vi "test Get-Set-Get AIM Hardware Parameters.vi"(8 "error in":errorcluster, 11 "TestCase in":refnum<class "Scripting.lvclass">) -> (0 "error out":errorcluster, 3 "TestCase out":refnum<class "Scripting.lvclass">)   [LabVIEW 2020, in "Scripting.lvclass"]
uses:
  Scripting.lvclass
  <vilib>/addons/_JKI Toolkits/VI Tester/TestCase.llb/TestCase.lvclass
  Scripting/AIM MIL-STD-1553 Scripting.lvlib
  Shared/Initialization Method.ctl
  Shared/AIM Hardware Parameters.ctl
  Shared/Coupling Mode.ctl
  Shared/Bus Selection.ctl
  Shared/Timing Mode.ctl
  C:/Program Files (x86)/National Instruments/LabVIEW 2020/vi.lib/addons/_JKI Toolkits/VI Tester/TestCase.llb/TestCase.lvclass
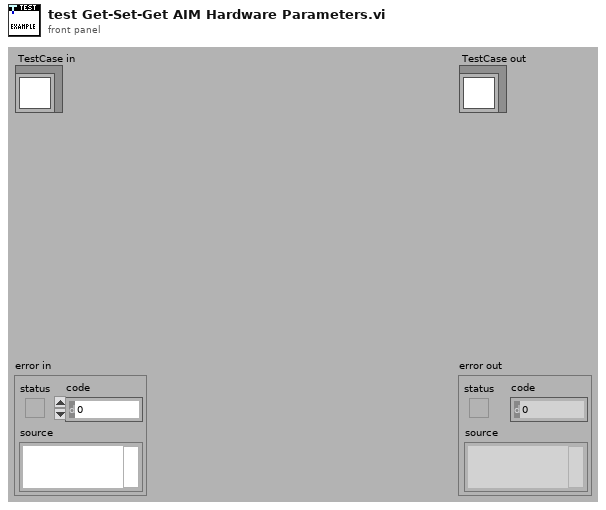
[diagram p1: front panel]
types:
  T1 = typedef "AIM Hardware Parameters.ctl" = cluster{"initialization method":T2, "card number":i32, "pxi slot number":i32, "biu number":i32, "bus selection":T3, "coupling mode":T4, "timing mode":T5}
  T2 = typedef "Initialization Method.ctl" = enum16{"PXI Slot Number", "Card Number"}
  T3 = typedef "Bus Selection.ctl" = enum16{"Both", "Primary", "Secondary"}
  T4 = typedef "Coupling Mode.ctl" = enum16{"Isolated Onboard Termination", "Transformer Coupled", "Direct Coupled", "External with Onboard Termination", "Onboard Digital Wrap-around"}
  T5 = typedef "Timing Mode.ctl" = enum16{"Disabled (Relative Timestamps)", "IRIG (Internal System Time)", "IRIG (External Timing Source)"}
  T6 = typedef "Custom Device API.lvlib/Custom Device Item Ref.ctl" = u64
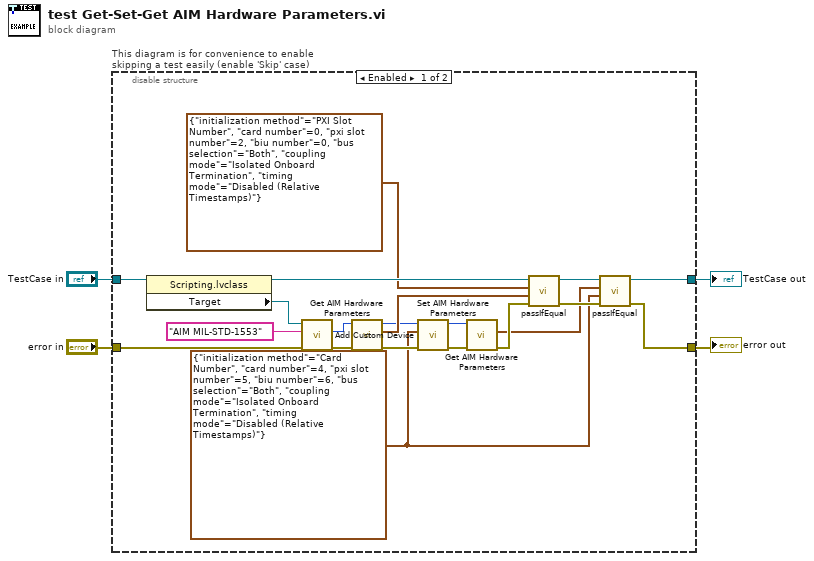
[diagram p0: block diagram]
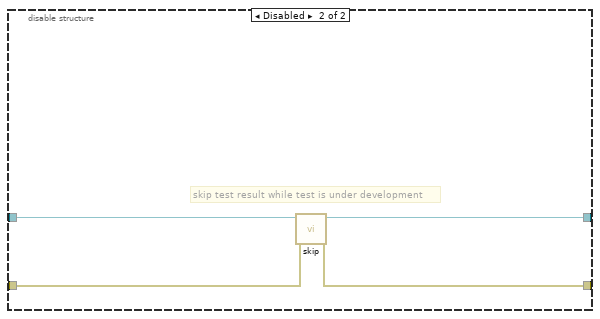
[diagram p2: hidden frame]
diagram:
  n1 = disable-structure "This diagram is for convenience to enable skipping a test easily (enable 'Skip' case)" shown="Enabled" {
    disable-tunnel: "TestCase in" -> [w20 w28]
    disable-tunnel: [w22 w26] -> w1
    disable-tunnel: [w21 w27] -> w3
    disable-tunnel: "error in" -> [w24 w25]
    frame Enabled {
      w6 = T1 {"initialization method"=enum."Card Number", "card number"=4, "pxi slot number"=5, "biu number"=6, "bus selection"=enum."Both", "coupling mode"=enum."Isolated Onboard Termination", "timing mode"=enum."Disabled (Relative Timestamps)"} ("device parameters")
      n2 = property class="Scripting.lvclass"(reference=w20) -> (reference out=w18:refnum<class "Scripting.lvclass">, "Target"=w19:refnum<k24>)  [unwired: 1 in, 1 out]
      n3 = call "Add Custom Device.vi"("error in"=w24, "custom device name"="AIM MIL-STD-1553" ("name"), "target"=w19) -> ("error out"=w17:errorcluster, "custom device"=w16:T6)  [unwired: 6 in, 1 out]
      n4 = call "Get AIM Hardware Parameters.vi"("error in"=w17, "custom device"=w16) -> ("error out"=w13:errorcluster, "aim hardware parameters"=w15:T1, "custom device out"=w14:T6)  [unwired: 7 in]
      n5 = call "Set AIM Hardware Parameters.vi"("error in"=w13, "aim hardware parameters"=w6, "custom device"=w14) -> ("error out"=w12:errorcluster, "custom device out"=w11:T6)  [unwired: 7 in]
      n6 = call "Get AIM Hardware Parameters.vi"("error in"=w12, "custom device"=w11) -> ("error out"=w10:errorcluster, "aim hardware parameters"=w7:T1)  [unwired: 7 in, 1 out]
      n7 = call-dynamic "passIfEqual.vi"("error in (no error)"=w10, "y"=w15, "x"=T1 {"initialization method"=enum."PXI Slot Number", "card number"=0, "pxi slot number"=2, "biu number"=0, "bus selection"=enum."Both", "coupling mode"=enum."Isolated Onboard Termination", "timing mode"=enum."Disabled (Relative Timestamps)"} ("device parameters"), "TestCase in"=w18) -> ("error out"=w8:errorcluster, "TestCase out"=w9:refnum<class "Scripting.lvclass">)  [unwired: 6 in]
      n8 = call-dynamic "passIfEqual.vi"("error in (no error)"=w8, "y"=w6, "x"=w7, "TestCase in"=w9) -> ("error out"=w21:errorcluster, "TestCase out"=w22:refnum<class "Scripting.lvclass">)  [unwired: 6 in]
    }
    frame Disabled {
      # "skip test result while test is under development"
      n9 = call <vilib>:"skip.vi"("error in (no error)"=w25, "TestCase in"=w28) -> ("error out"=w27:errorcluster, "TestCase out"=w26:refnum<class "Scripting.lvclass">)  [unwired: 8 in]
    }
  }
  "error out" <- w3
  "TestCase out" <- w1
